vi "GetFrame.vi"(8 "error in (no error)":errorcluster, 11 "HamaCam in":refnum<class "HamaCam.lvclass">) -> (0 "error out":errorcluster, 3 "HamaCam out":refnum<class "HamaCam.lvclass">)   [LabVIEW 2023, in "HamaCam.lvlib" / "HamaCam.lvclass"]
uses:
  HamaCam.lvclass
  HamaCam.lvclass/HamaCam.ctl
  Interfaces/AbstractInstrumentClasses/Cameras_LV/CameraDAQ Messages/GrabFrame Msg/GrabFrame Msg.lvclass
  <vilib>/ActorFramework/Actor/Actor.lvclass
  Applications/National Instruments/LabVIEW 2023 64-bit/vi.lib/ActorFramework/Actor/Actor.lvclass
  Users/alexandrosspiliotis/Documents/LV_DAQ_Project/ConcreteClasses/ConcreteInstrumentClasses/CameraClasses/Hama_LV/HamaCam/HamaCam/HamaCam.lvclass
  Users/alexandrosspiliotis/Documents/LV_DAQ_Project/Interfaces/AbstractInstrumentClasses/Cameras_LV/CameraInterface/CameraInterface.lvclass
  Users/alexandrosspiliotis/Documents/LV_DAQ_Project/Interfaces/InitDeinitInterface/InitDeinit/InitDeinit.lvclass
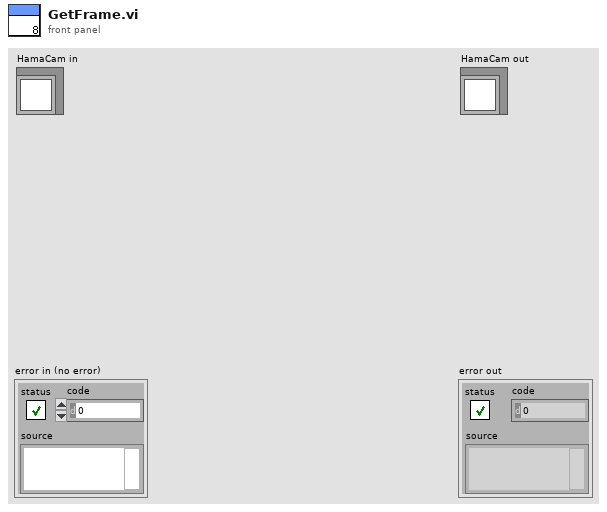
[diagram p1: front panel]
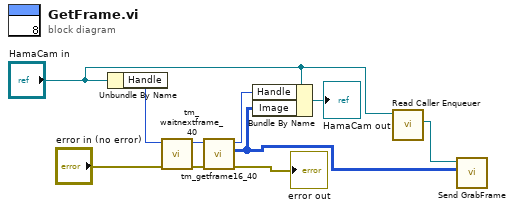
[diagram p0: block diagram]
diagram:
  n1 = Unbundle By Name("HamaCam in") -> ("Handle"=w8:u32)
  n2 = call "tm_waitnextframe_40.vi"("error in (no error)"="error in (no error)", "Handle in"=w8) -> ("error out"=w6:errorcluster, "Handle out"=w9:u32)  [unwired: 6 in, 2 out]
  n3 = call "tm_getframe16_40.vi"("error in (no error)"=w6, "Handle in"=w9) -> ("error out"=→"error out":errorcluster, "Data"=w3:u16[][], "Handle out"=w10:u32)  [unwired: 6 in, 1 out]
  n4 = Bundle By Name(cluster="HamaCam in", "Handle"=w10, "Image"=w3) -> (→"HamaCam out":refnum<class "HamaCam.lvclass">)
  n5 = call <vilib>:"Read Caller Enqueuer.vi"("Actor"="HamaCam in") -> ("Caller Enqueuer"=w2:refnum<class "Message Enqueuer.lvclass">)  [unwired: 10 in]
  n6 = call "Send GrabFrame.vi"("Image"=w3, "Message Enqueuer"=w2) -> ()  [unwired: 8 in, 2 out]
